vi "Self Configure.vi"(8 "error in":errorcluster, 11 "PRM in":refnum<class "PRM.lvclass">) -> (0 "error out":errorcluster, 3 "PRM out":refnum<class "PRM.lvclass">)   [LabVIEW 2019, in "PRM.lvlib" / "PRM.lvclass"]
doc: "Children of Instruments must override this routine and call the parent method. \nThis routine is implemented to allow each instrument to read its specific configuration keys and implement any default configuration settings.\n\nThis routine already calls Connect and Self Test Routines."
uses:
  Library/PRM.lvclass
  builds/Instruments/Instruments.lvlibp/Library/Instruments.lvclass
  builds/Tools/Config.lvlibp/Config.lvclass
  C:/Users/Public/Documents/Development/builds/Tools/Config.lvlibp/Config.lvclass
  Custom Controls/Configuration Keys.ctl
  Custom Controls/Operational Mode.ctl
panel:
  in  "Mode":T1
  in  "Configuration Keys":T2
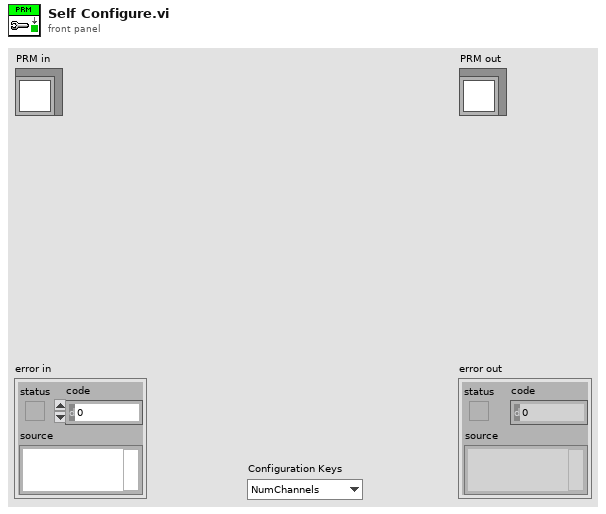
[diagram p1: front panel]
types:
  T1 = typedef "PRM.lvlib/PRM.lvclass/Operational Mode.ctl" = enum16{"RESISTANCE", "TEMPERATURE", "POTENTIOMETER"}
  T2 = typedef "PRM.lvlib/PRM.lvclass/Configuration Keys.ctl" = enum16{"NumChannels", "OperationMode"}
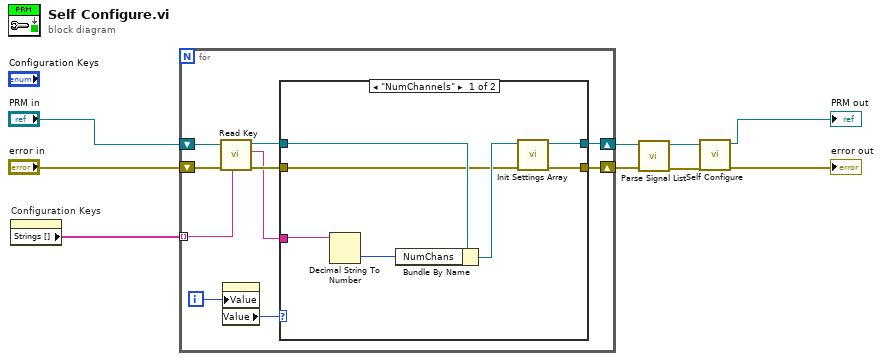
[diagram p0: block diagram]
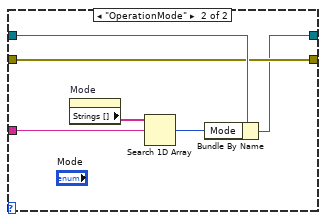
[diagram p2: hidden frame]
diagram:
  n1 = property on="Configuration Keys" class="Enum (strict)"() -> ("Strings []"=w5:string[])  [unwired: 2 in, 2 out]
  n2 = for {
    tunnel: w5 -> [w13] mode=indexing
    shift-right: [w10] -> w3
    shift-left: "PRM in" -> [w15]
    shift-right: [w11] -> w1
    shift-left: "error in" -> [w17]
    i -> [w19]
    n3 = call "Read Key.vi"("Key Name"=w13, "error in"=w17, "Config in"=w15) -> ("error out"=w16:errorcluster, "Key Value"=w12:string, "Config out"=w14:refnum<class "PRM.lvclass">)  [unwired: 6 in]
    n4 = property on="Configuration Keys" class="Enum (strict)"("Value"=w19) -> ("Value"=w18:T2)  [unwired: 2 in, 2 out]
    n5 = case shown="\"NumChannels\"" w18 {
      tunnel: w16 -> [w22 w31]
      tunnel: w14 -> [w26 w32]
      tunnel: w12 -> [w25 w29]
      tunnel: [w21 w31] -> w11
      tunnel: [w20 w30] -> w10
      frame "NumChannels" {
        n6 = Decimal String To Number(string=w25) -> (number=w24:i32)  [unwired: 2 in, 1 out]
        n7 = Bundle By Name(cluster=w26, "NumChans"=w24) -> (w23:refnum<class "PRM.lvclass">)
        n8 = call "Init Settings Array.vi"("error in (no error)"=w22, "PRM in"=w23) -> ("error out"=w21:errorcluster, "PRM out"=w20:refnum<class "PRM.lvclass">)  [unwired: 8 in]
      }
      frame "OperationMode" {
        n9 = property on="Mode" class="Enum (strict)"() -> ("Strings []"=w28:string[])  [unwired: 2 in, 2 out]
        n10 = Search 1D Array(1D array=w28, element=w29) -> (index of element=w27:i32)  [unwired: 1 in]
        n11 = Bundle By Name(cluster=w32, "Mode"=w27) -> (w30:refnum<class "PRM.lvclass">)
      }
    }
  }
  n12 = call "Parse Signal List.vi"("error in"=w1, "PRM in"=w3) -> ("error out"=w7:errorcluster, "PRM out"=w6:refnum<class "PRM.lvclass">)  [unwired: 8 in]
  n13 = call-parent "Self Configure.vi"("error in"=w7, "Instruments in"=w6) -> ("error out"=→"error out":errorcluster, "Instruments out"=→"PRM out":refnum<class "PRM.lvclass">)  [unwired: 8 in]
